vi "Auto Catapult Mode.vi"() -> (13 "States":T1, 14 "high 1":bool, 15 "high 2":bool, 16 "high 3":bool, 17 "high 4":bool, 18 "Jank Boi":bool, 19 "Ball Security":bool)   [LabVIEW 2015]
uses:
  Common Code/Catapult/Catapult State.ctl
  Common Code/Intake Commands.ctl
  Common Code/Change Detect Int.vi
  Robot Global Data.vi
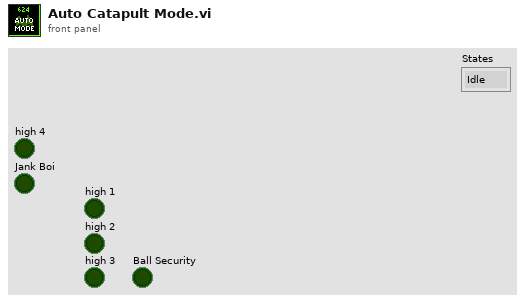
[diagram p1: front panel]
types:
  T1 = typedef "Catapult State.ctl" = enum16{"Idle", "Warmup", "Shoot"}
  T2 = typedef "Intake Commands.ctl" = enum16{"Zero", "Unload", "Load", "Drop low", "Idle"}
  T3 = typedef "Dashboard Control Data.ctl" = cluster{"Encoder Control":T4, "Steer PID output":cluster{"output high":dbl, "output low":dbl}, " Steer PID gains":cluster{"proportional gain (Kc)":dbl, "integral time (Ti, min)":dbl, "derivative time (Td, min)":dbl}, "Drivetrain Settings":T5, "Vision Packet":T6, "Dashboard Drivetrain Command":T7, "Info/Command Cluster":T9, "Ball Vision Packet":T10, "Intake Presets":T12, "Intake Encoder Control":T14, "Goal Output Range":cluster{"output high":dbl, "output low":dbl}, "Enabled Systems":T15, "Auton Presets":T16, "Pressure M":dbl, "Pressure B":dbl, "Vision Timeout":dbl, "Auto-Shift":T17, "Catapult Setpoints":T18, "Climb Presets":T19}
  T4 = typedef "Encoder Control.ctl" = cluster{"Right Tick Constant":dbl, "Left Tick Constant":dbl, "Reset?":bool, "Y Dist":cluster{"PID gains":cluster{"proportional gain (Kc)":dbl, "integral time (Ti, min)":dbl, "derivative time (Td, min)":dbl}}, "Y Stop Thresh":dbl, "Y Stop Speed":dbl}
  T5 = typedef "Drivetrain Settings.ctl" = cluster{"Gyro Tolerance":dbl, "Throttle Ramp (ms)":dbl, "Kv":dbl, "Ka":dbl, "Feed Forward P":dbl, "Feed Forward D":dbl, "Goal Vision PID gains":cluster{"proportional gain (Kc)":dbl, "integral time (Ti, min)":dbl, "derivative time (Td, min)":dbl}, "Goal Detection Window":dbl, "Creep Rate":dbl, "Vision Throttle Threshold":dbl, "Min Turn Output":dbl, "Left Batter Angle":dbl, "Right Batter Angle":dbl}
  T6 = typedef "Goal Vision Packet.ctl" = cluster{"Distance":dbl, "Center X":dbl, "Center Y":dbl, "Found Target?":bool, "Robot Center":dbl, "Angle":dbl}
  T7 = typedef "Dashboard Drivetrain Command.ctl" = cluster{"Drivetrain Vision":T8}
  T8 = typedef "Drivetrain Vision.ctl" = cluster{"Goal Window":dbl, "Ball Window":dbl}
  T9 = typedef "Ball Tracking Command Cluster.ctl" = cluster{"Distance to Ball":dbl, "Desired Angle":dbl, "Command":enum16{"Turn to Ball", "Turn to Angle", "Get Distance"}, "Pixels from Center":dbl}
  T10 = typedef "Ball Vision Packet.ctl" = cluster{"Ball Detected?":bool, "Distance to Ball":dbl, "Desired Angle":dbl, "Pixels from Center":dbl, "Tracking mode":T11}
  T11 = typedef "Tracking Mode.ctl" = enum16{"Turn to Ball", "Turn to Angle"}
  T12 = typedef "Intake Presets.ctl" = cluster{"Intake Speed":dbl, "Outake Speed":dbl, "Angle Speed":dbl, "Angle Tolerance":dbl, "Encoder Scale":dbl, "Load Height":dbl, "Output Range":T13, "MaxCurrent":dbl, "Idle Height":dbl, "Max Height":dbl, "Reset Encoders?":bool, "PID gains":cluster{"proportional gain (Kc)":dbl, "integral time (Ti, min)":dbl, "derivative time (Td, min)":dbl}, "Drop Low Height ":dbl, "Rotation Power Max/Min":dbl, "Reset Delay":dbl, "Current Trip Delay":dbl}
  T13 = typedef "Drivetrain Output Range.ctl" = cluster{"output high":dbl, "output low":dbl}
  T14 = typedef "IntakeEcoderControl.ctl" = cluster{"Arm Tick Constant":dbl, "Reset?":bool, "Y Dist":cluster{"PID gains":cluster{"proportional gain (Kc)":dbl, "integral time (Ti, min)":dbl, "derivative time (Td, min)":dbl}}, "Y Stop Thresh":dbl, "Y Stop Speed":dbl}
  T15 = typedef "Enabled Systems.ctl" = cluster{"Shoot":bool, "Intake":bool, "DT":bool, "Gyro":bool, "100ms":bool, "US":bool}
  T16 = typedef "Autonomous Presets.ctl" = cluster{"Pitch Limit":dbl, "Roll Limit":dbl, "Start Position":dbl, "Cross Position":dbl}
  T17 = typedef "Auto Shift Cluster.ctl" = cluster{"Delay":dbl, "Speed Thresh":dbl, "Upshift Accel":dbl, "Upshift Throttle":dbl, "Upshift Throttle Accel":dbl, "Downshift Throttle":dbl, "Downshift Throttle Accel":dbl, "Pressure Threshold":dbl}
  T18 = typedef "Catapult Presets.ctl" = cluster{"Intake Danger Height":dbl, "Ball Security Delay ":dbl, "High PSI Minimum":dbl, "Shot Finish Delay":dbl, "Low PSI Minimum":dbl, "Idle Ball Security Wait ":dbl}
  T19 = typedef "Climb Presets.ctl" = cluster{"Winch Speed":dbl, "Wait until Fire":dbl, "Wait until Winch":dbl, "Wait until Stop":dbl}
  T20 = typedef "Catapult Command Cluster.ctl" = cluster{"States":T21, "Mode":T22, "Override IR":bool, "Shoot Mode":T23, "Ball Loaded?":bool, "High Pressure?":bool, "Shoot?":bool, "Flashlight ":bool}
  T21 = typedef "Catapult Auto Commands.ctl" = enum16{"Idle", "Warmup", "Shoot"}
  T22 = typedef "Catapult Modes.ctl" = enum16{"Auto"}
  T23 = typedef "Shoot Mode.ctl" = enum16{"Outer", "Batter"}
  T24 = typedef "Intake Status Cluster.ctl" = cluster{"Roller Power":dbl, "Angle Power":dbl, "Intake Mode":T25, "Rollers Active?":bool, "Current Height":dbl, "Target Height":dbl, "Encoder Raw Position":dbl, "Forward Tripped?":bool, "Backward Tripped?":bool, "Override IR?":bool, "Intake State":T2}
  T25 = typedef "Intake Mode.ctl" = enum16{"Manual", "Safe", "Auto"}
  T26 = typedef "Drivetrain Status Cluster.ctl" = cluster{"Modes":T27, "Y (Throttle)":dbl, "X (Steer)":dbl, "Gyro In Range?":bool, "Distance Drive Finished?":bool, "Stop Eject Lockout":bool, "Dist Drive Status":T28, "Y Target":dbl, "Heading Target":dbl, "Vision Target Aligned?":bool}
  T27 = typedef "Drivetrain Modes.ctl" = enum16{"Gyro Steer", "Manual", "Goal Vision Targeting", "PID Distance Drive", "Hybrid"}
  T28 = typedef "Dist Drive Status.ctl" = cluster{"Y In Range":bool, "X In Range":bool, "Gyro In Range":bool, "Y Dist":dbl, "X Dist":dbl, "Gyro":dbl}
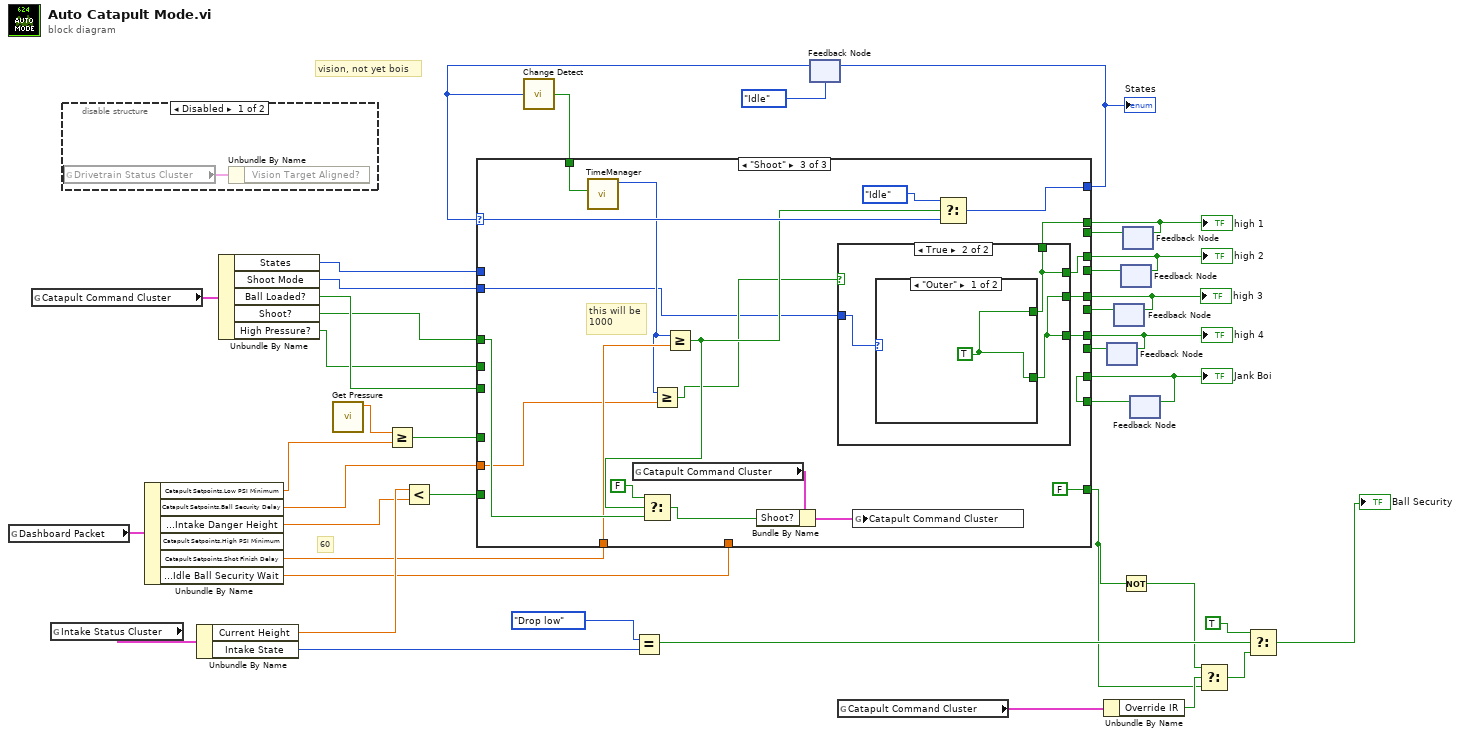
[diagram p0: block diagram]
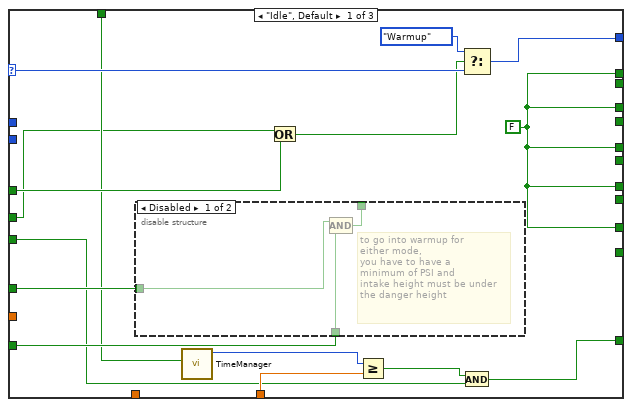
[diagram p2: hidden frame]
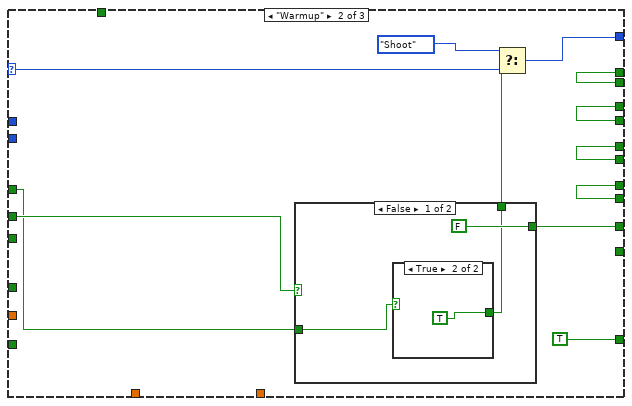
[diagram p4: hidden frame]
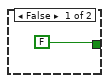
[diagram p5: hidden frame]
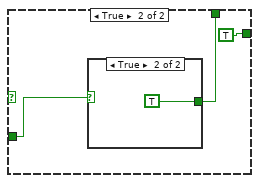
[diagram p6: hidden frame]
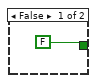
[diagram p7: hidden frame]
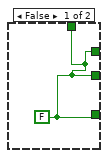
[diagram p8: hidden frame]
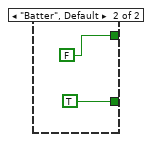
[diagram p9: hidden frame]
diagram:
  # "60"
  # "vision, not yet bois"
  n1 = global read "Robot Global Data.vi" "Dashboard Packet"() -> (w40:T3)
  n2 = global read "Robot Global Data.vi" "Catapult Command Cluster"() -> (w36:T20)
  n3 = global read "Robot Global Data.vi" "Intake Status Cluster"() -> (w39:T24)
  n4 = disable-structure shown="Disabled" {
    frame Disabled {
      n5 = global read "Robot Global Data.vi" "Drivetrain Status Cluster"() -> (w42:T26)
      n6 = Unbundle By Name(w42) -> ()  [unwired: 1 out]
    }
    frame Enabled {
    }
  }
  n7 = Unbundle By Name(w40) -> ("Catapult Setpoints.Low PSI Minimum"=w16:dbl, "Catapult Setpoints.Ball Security Delay"=w14:dbl, "Catapult Setpoints.Intake Danger Height"=w20:dbl, "Catapult Setpoints.Shot Finish Delay"=w18:dbl, "Catapult Setpoints.Idle Ball Security Wait"=w11:dbl)  [unwired: 1 out]
  n8 = Unbundle By Name(w39) -> ("Current Height"=w21:dbl, "Intake State"=w9:T2)
  n9 = Unbundle By Name(w36) -> ("States"=w22:T21, "Shoot Mode"=w37:T23, "Ball Loaded?"=w13:bool, "Shoot?"=w12:bool, "High Pressure?"=w10:bool)
  n10 = call "Get Pressure.vi"() -> ("Pressure"=w17:dbl)  [unwired: 10 in, 1 out]
  n11 = Greater Or Equal?(x=w17, y=w16) -> (x >= y?=w15:bool)
  n12 = Less?(x=w21, y=w20) -> (x < y?=w19:bool)
  n13 = Equal?(x=Intake_Commands."Drop low" ("Intake State"), y=w9) -> (x = y?=w7:bool)
  n14 = feedback #1(Catapult_State."Idle") -> (w38:T1)
  n15 = call-poly "Change Detect.vi"("In"=w38) -> ("Changed?"=w31:bool)
  n16 = global read "Robot Global Data.vi" "Catapult Command Cluster"() -> (w35:T20)
  n17 = Unbundle By Name(w35) -> ("Override IR"=w3:bool)
  n18 = feedback #2() -> (w23:bool)  [unwired: 1 in]
  n19 = feedback #3() -> (w25:bool)  [unwired: 1 in]
  n20 = feedback #4() -> (w27:bool)  [unwired: 1 in]
  n21 = feedback #5() -> (w29:bool)  [unwired: 1 in]
  n22 = feedback #6() -> (w33:bool)  [unwired: 1 in]
  n23 = case shown="\"Shoot\"" w38 {
    selector: w38 -> [w54 w71 w99]
    tunnel: [w45 TRUE FALSE] -> w1
    tunnel: w37 -> [_ _ w88]
    tunnel: [w57 w62 w103] -> w34
    tunnel: w33 -> [_ _ w103]
    tunnel: w22 -> [_ _ _]
    tunnel: [w56 w70 w101] -> w32
    tunnel: w31 -> [w49 _ w102]
    tunnel: [w57 w69 w85] -> w30
    tunnel: [w57 w68 w84] -> w28
    tunnel: [w57 w67 w86] -> w26
    tunnel: [w57 w66 w87] -> w24
    tunnel: w29 -> [_ w69 _]
    tunnel: w27 -> [_ w68 _]
    tunnel: w25 -> [_ w67 _]
    tunnel: w23 -> [_ w66 _]
    tunnel: w13 -> [w46 _ _]
    tunnel: w19 -> [w51 _ _]
    tunnel: w18 -> [_ _ w92]
    tunnel: w15 -> [w52 _ _]
    tunnel: w14 -> [_ _ w90]
    tunnel: w12 -> [w53 w64 w94]
    tunnel: w11 -> [w47 _ _]
    tunnel: w10 -> [w44 w65 _]
    frame "Idle", Default {
      w57 = FALSE
      n24 = disable-structure shown="Disabled" {
        disable-tunnel: w52 -> [w60 _]
        disable-tunnel: w51 -> [w59 _]
        disable-tunnel: [w58 _] -> _
        frame Disabled {
          # "to go into warmup for \neither mode, \nyou have to have a \nminimum of PSI and \nintake height must be under\nthe danger height"
          n25 = Compound Arithmetic op=AND(w60, w59) -> (w58:bool)
        }
        frame Enabled {
        }
      }
      n26 = call "TimeManager.vi"("Reset?"=w49) -> ("Time Since Reset"=w48:u32)  [unwired: 9 in, 1 out]
      n27 = Or(x=w44, y=w53) -> (x .or. y?=w50:bool)
      n28 = Greater Or Equal?(x=w48, y=w47) -> (x >= y?=w43:bool)
      n29 = Select(t=Catapult_State."Warmup", s=w50, f=w54) -> (s? t:f=w56:T1)
      n30 = And(x=w43, y=w46) -> (x .and. y?=w45:bool)
    }
    frame "Warmup" {
      n31 = case shown="False" w65 {
        tunnel: w64 -> [w74 w80]
        tunnel: [w73 w79] -> w63
        tunnel: [FALSE TRUE] -> w62
        frame False {
          n32 = case shown="True" w74 {
            tunnel: [FALSE TRUE] -> w73
            frame False {
            }
            frame True {
            }
          }
        }
        frame True {
          n33 = case shown="True" w80 {
            tunnel: [FALSE TRUE] -> w79
            frame False {
            }
            frame True {
            }
          }
        }
      }
      n34 = Select(t=Catapult_State."Shoot", s=w63, f=w71) -> (s? t:f=w70:T1)
    }
    frame "Shoot" {
      # "this will be\n1000"
      n35 = call "TimeManager.vi"("Reset?"=w102) -> ("Time Since Reset"=w91:u32)  [unwired: 9 in, 1 out]
      n36 = global read "Robot Global Data.vi" "Catapult Command Cluster"() -> (w98:T20)
      n37 = Greater Or Equal?(x=w91, y=w90) -> (x >= y?=w89:bool)
      n38 = Greater Or Equal?(x=w91, y=w92) -> (x >= y?=w93:bool)
      n39 = Select(t=FALSE, s=w93, f=w94) -> (s? t:f=w95:bool)
      n40 = Bundle By Name(cluster=w98, "Shoot?"=w95) -> (w97:T20)
      n41 = case shown="True" w89 {
        tunnel: w88 -> [_ w107]
        tunnel: [w104 w106] -> w87
        tunnel: [w104 w106] -> w86
        tunnel: [w104 w105] -> w84
        tunnel: [w104 w105] -> w85
        frame False {
          w104 = FALSE
        }
        frame True {
          n42 = case shown="\"Outer\"" w107 {
            tunnel: [w108 TRUE] -> w106
            tunnel: [w108 FALSE] -> w105
            frame "Outer" {
              w108 = TRUE
            }
            frame "Batter", Default {
            }
          }
        }
      }
      n43 = global write "Robot Global Data.vi" "Catapult Command Cluster"(w97) -> ()
      n44 = Select(t=Catapult_State."Idle", s=w93, f=w99) -> (s? t:f=w101:T1)
    }
  }
  "high 1" <- w30
  "high 2" <- w28
  "high 3" <- w26
  "high 4" <- w24
  "Jank Boi" <- w34
  "States" <- w32
  n45 = feedback-in #1(w32) -> ()
  n46 = feedback-in #2(w24) -> ()
  n47 = feedback-in #3(w26) -> ()
  n48 = feedback-in #4(w28) -> ()
  n49 = Not(x=w1) -> (.not. x?=w2:bool)
  n50 = feedback-in #5(w30) -> ()
  n51 = feedback-in #6(w34) -> ()
  n52 = Select(t=w2, s=w3, f=w1) -> (s? t:f=w4:bool)
  n53 = Select(t=TRUE, s=w7, f=w4) -> (s? t:f=→"Ball Security":bool)
